vi "Read Instance ID.vi"(8 "error in":errorcluster, 11 "EthernetIP Channel in":refnum<class "EIP Tags Channel.lvclass">) -> (0 "error out":errorcluster, 2 "Instance ID":u32, 3 "EthernetIP Channel out":refnum<class "EIP Tags Channel.lvclass">)   [LabVIEW 2013, in "EIP Tags Channel.lvclass"]
uses:
  EIP Tags Channel.lvclass
  EIP Tags Channel.lvclass/EIP Tags Channel.ctl
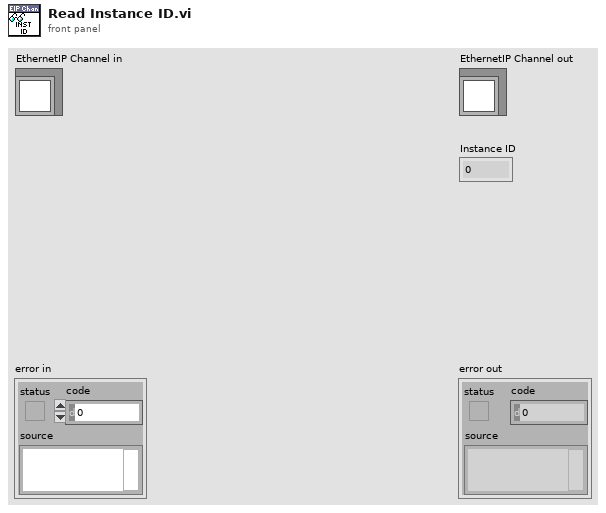
[diagram p1: front panel]
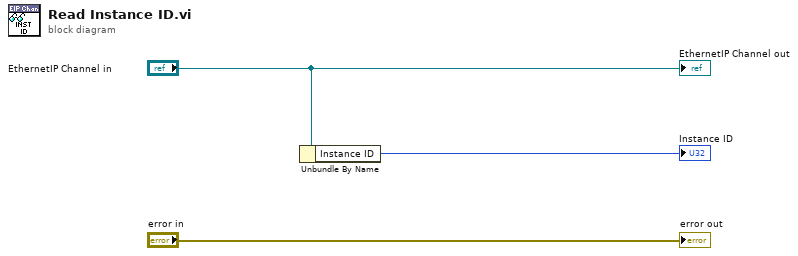
[diagram p0: block diagram]
diagram:
  n1 = Unbundle By Name("EthernetIP Channel in") -> ("Instance ID"=→"Instance ID":u32)
  "error out" <- "error in"
  "EthernetIP Channel out" <- "EthernetIP Channel in"
